vi "Bind to Name - Non Serializable Class - Returns Empty String.vi"() -> ()   [LabVIEW 2017, in "JSON Serializable Binder Tests.lvlib"]
uses:
  JSON Serializable Binder Tests.lvlib
  JSON Serializable Binder/JSON Serializable Binder.lvclass
  <vilib>/addons/_JKI Toolkits/Caraya/classes/Assert/Assert Equal Value_Variant.vi
  <vilib>/addons/_JKI Toolkits/Caraya/classes/Test/Test.lvclass
  <vilib>/addons/_JKI Toolkits/Caraya/classes/Assert/Assert.lvclass
panel:
  out "error out":errorcluster
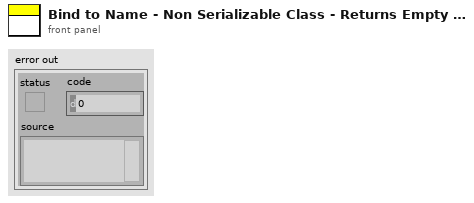
[diagram p1: front panel]
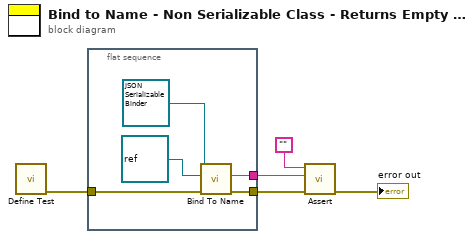
[diagram p0: block diagram]
diagram:
  n1 = call <vilib>:"Define Test.vi"() -> ("error out"=w4:errorcluster)  [unwired: 11 in]
  n2 = flat-sequence {
    tunnel: [w6] -> w5
    tunnel: w4 -> [w7]
    tunnel: [w8] -> w2
    frame #0 {
      n3 = call-dynamic "Bind To Name.vi"("error in (no error)"=w7, "Type"=refnum<class> refnum, "JSON Serializable Binder in"=refnum<class "JSON Serializable Binder.lvclass"> refnum ("JSON Serializable Binder.lvclass")) -> ("error out"=w6:errorcluster, "Type Name"=w8:string)  [unwired: 6 in, 1 out]
    }
  }
  n4 = call-poly <vilib>:"Assert.vi"("error in (no error)"=w5, "Y"=w2, "X"="") -> ("error out"=→"error out":errorcluster)  [unwired: 8 in]
